vi "New Queue Log.vi"(6 "queue (default: new)":refnum<queue>, 7 "context":string, 8 "error in (no error)":errorcluster, 10 "level":T1 items=["OFF"=0, "FATAL"=100, "ERROR"=200, "WARN"=300, "INFO"=400, "DEBUG"=500, "TRACE"=600, "ALL"=65535]) -> (0 "error out":errorcluster, 1 "queue out":refnum<queue>, 3 "Queue Log Provider":refnum<data-value>)   [LabVIEW 2019, in "LVCOOOP.lvlib" / "Support API.lvlib" / "Queue Log Provider.lvclass"]
uses:
  Queue Log Provider.lvclass
  Log Service/public/level.ctl
  Log Service/Log Service.lvclass
  impl/log_message.ctl
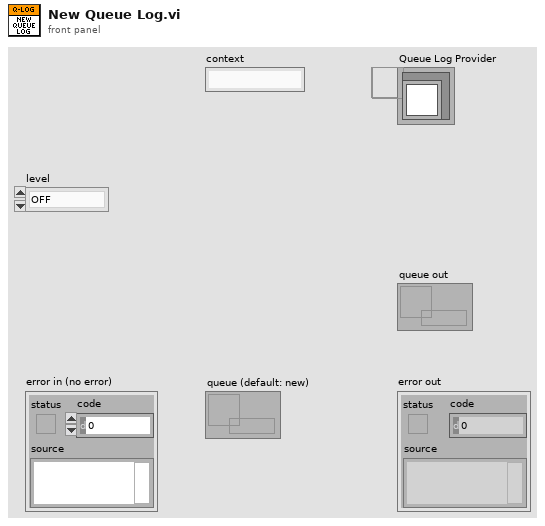
[diagram p1: front panel]
types:
  T1 = typedef "LVCOOOP.lvlib/Support API.lvlib/Log Service.lvclass/level.ctl" = u16
  T2 = typedef "LVCOOOP.lvlib/Support API.lvlib/Queue Log Provider.lvclass/log_message.ctl" = cluster{"Time Stamp":timestamp, "level":T1, "context":string, "message":string}
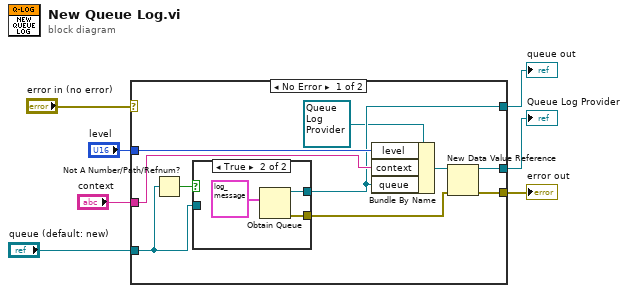
[diagram p0: block diagram]
diagram:
  n1 = case shown="No Error" "error in (no error)" {
    selector: "error in (no error)" -> [_ w23]
    tunnel: [w12 w23] -> w6
    tunnel: [w9 _] -> w5
    tunnel: "queue (default: new)" -> [w14 w22]
    tunnel: "context" -> [w16 _]
    tunnel: "level" -> [w15 _]
    tunnel: [w13 w22] -> w1
    frame No Error {
      n2 = Not A Number/Path/Refnum?(number/path/refnum=w14) -> (NaN/Path/Refnum?=w17:bool)
      n3 = case shown="True" w17 {
        tunnel: [w18 w20] -> w13
        tunnel: w14 -> [w18 _]
        tunnel: [_ w19] -> w11
        frame False {
        }
        frame True {
          n4 = Obtain Queue(element data type=T2 {"Time Stamp"=timestamp(0 s since 1904-01-01), "level"=0, "context"="", "message"=""} ("message")) -> (queue out=w20:refnum<queue>, error out=w19:errorcluster)  [unwired: 4 in, 1 out]
        }
      }
      n5 = Bundle By Name(cluster=refnum<class "Queue Log Provider.lvclass"> refnum ("Queue Log Provider in"), "level"=w15, "context"=w16, "queue"=w13) -> (w10:refnum<class "Queue Log Provider.lvclass">)
      n6 = New Data Value Reference(data value=w10, error in=w11) -> (data value reference=w9:refnum<data-value>, error out=w12:errorcluster)
    }
    frame Error {
    }
  }
  "error out" <- w6
  "Queue Log Provider" <- w5
  "queue out" <- w1
